vi "Clear-Receive.vi"(8 "错误输入":errorcluster caption="错误输入（无错误）", 10 "CANChannel":u32, 11 "DeviceType":T2=3 items=["PCI-CAN200"=7, "USB-CAN"=2, "USB-CAN200"=3]) -> (0 "错误输出":errorcluster, 1 "VCI_CAN_OBJ_R":T1={"ID"=96, 0, 0, 0, "TimeStamp"=0, "TimeFlag"=0, "SendType"=0, "RemoteFlag"=0, "ExternFlag"=0, "DataLen"=8, "Byte0"=0, "Byte1"=248, "Byte2"=17, "Byte3"=0, "Byte4"=0, "Byte5"=0, "Byte6"=0, "Byte7"=0, "Channel"=0, 77, 32} {"Byte7" format="%x"; "Byte6" format="%x"; "Byte5" format="%x"; "Byte4" format="%x"; "Byte3" format="%x"; "Byte2" format="%x"; "Byte1" format="%x"; "Byte0" format="%x"}, 2 "Result":bool=TRUE, 3 "DeviceTypeOut":u16(ring)=7 items=["PCI-CAN200"=7], 4 "帧数据":string, 5 "每次接收完时间":u32, 6 "data":string, 7 "ErrorSource":string)   [LabVIEW 2013]
uses:
  DevType.ctl
  VCI_CAN.dll
panel:
  out "VCI_CAN_OBJ_R 2":T1
  out "长度":string
  out "帧ID":string
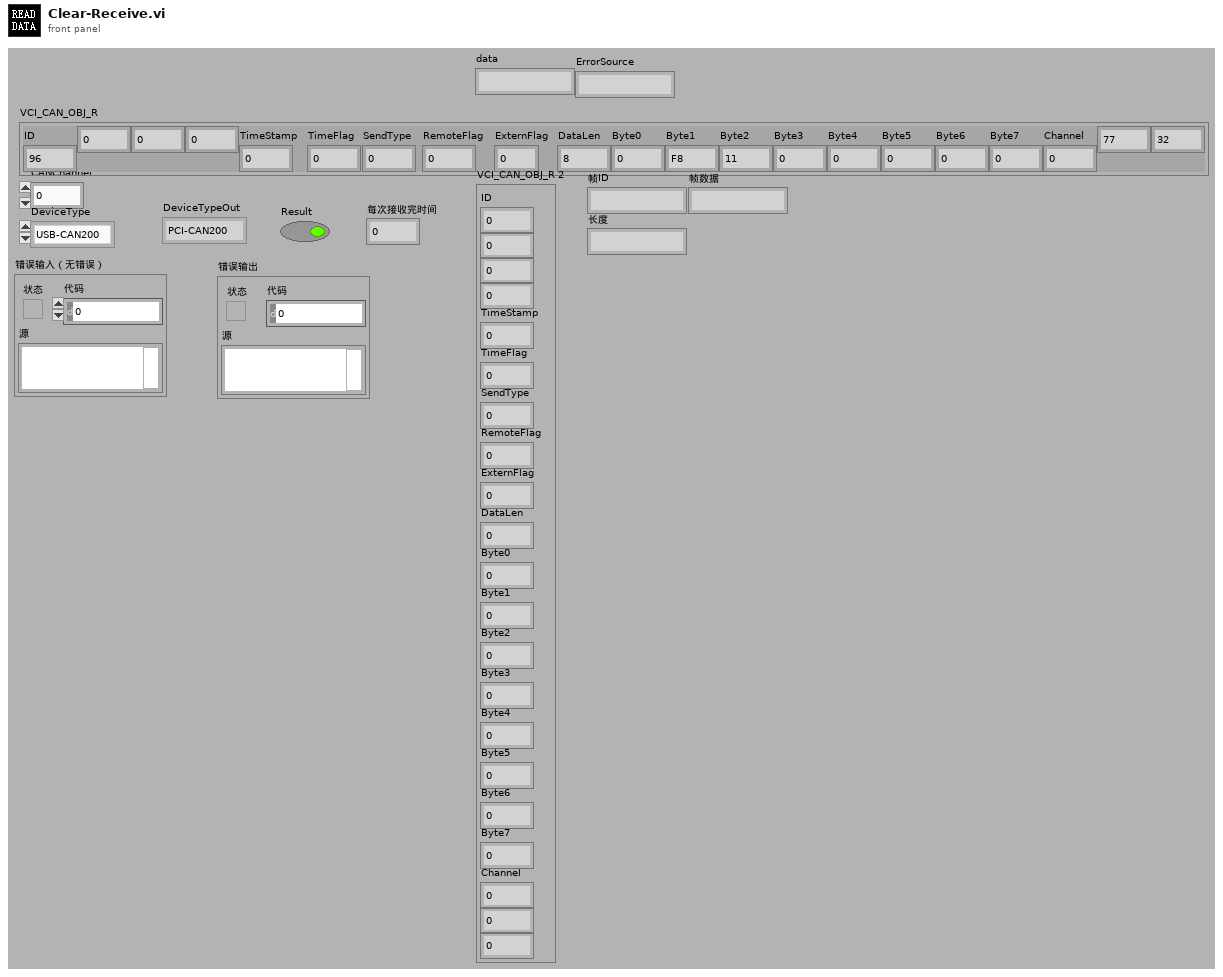
[diagram p1: front panel]
types:
  T1 = cluster{"ID":u8, u8, u8, u8, "TimeStamp":u32, "TimeFlag":u8, "SendType":u8, "RemoteFlag":u8, "ExternFlag":u8, "DataLen":u8, "Byte0":u8, "Byte1":u8, "Byte2":u8, "Byte3":u8, "Byte4":u8, "Byte5":u8, "Byte6":u8, "Byte7":u8, "Channel":u8, u8, u8}
  T2 = typedef "DevType.ctl" = u16
  T3 = cluster{"ID":u8, u8, u8, u8, "TimeStamp":u32, "TimeFlag":u8, "SendType":u8, "RemoteFlag":u8, "ExternFlag":u8, "DataLen":u8, u8, u8, u8, u8, u8, u8, u8, u8, u8, u8, u8}
  T4 = cluster{"ID":u8, u8, u8, u8, "TimeStamp":u32, "TimeFlag":u8, "SendType":u8, "RemoteFlag":u8, "ExternFlag":u8, "DataLen":u8, u8, u8, u8, u8, u8, u8, u8, u8, u8, u8, u8}[]
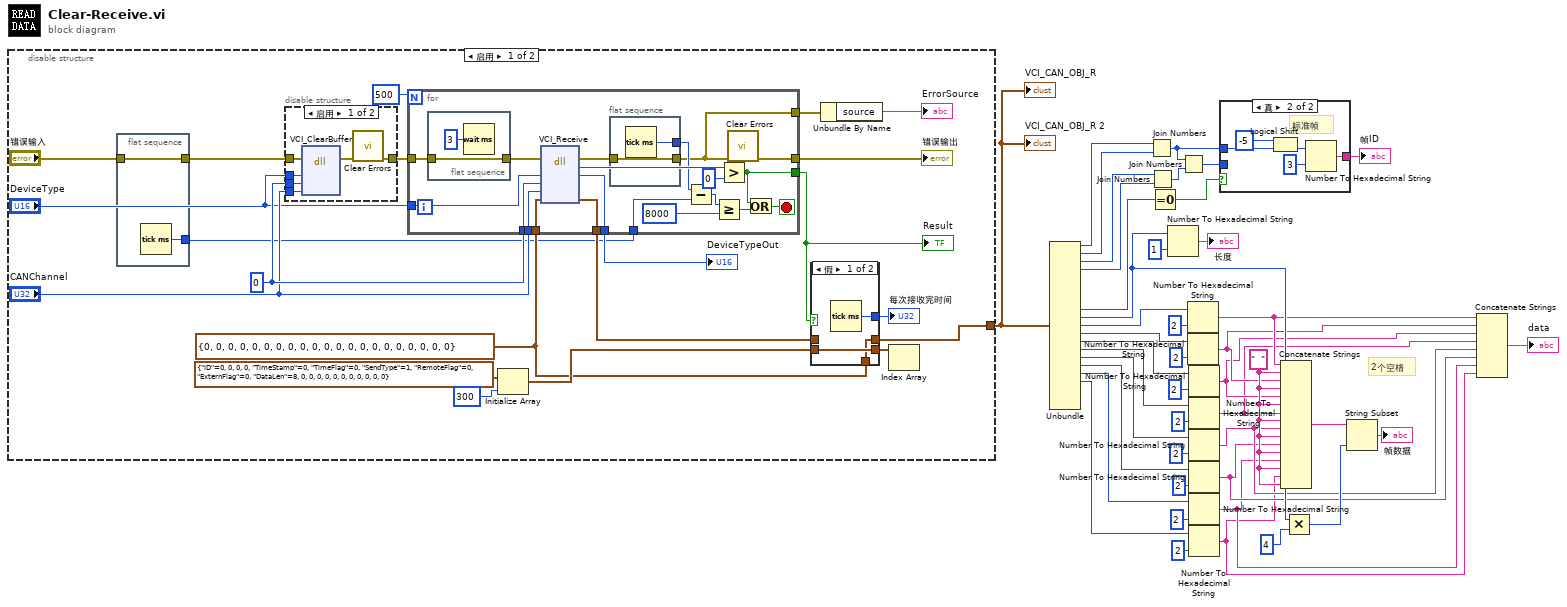
[diagram p0: block diagram]
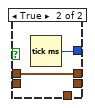
[diagram p3: hidden frame]
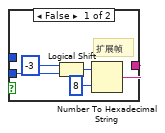
[diagram p5: hidden frame]
diagram:
  w23 = "  " ("字符串")
  # "2个空格"
  n1 = disable-structure shown="启用" {
    disable-tunnel: [w51 _] -> w10
    frame Enabled {
      w52 = T1 {"ID"=0, 0, 0, 0, "TimeStamp"=0, "TimeFlag"=0, "SendType"=0, "RemoteFlag"=0, "ExternFlag"=0, "DataLen"=0, "Byte0"=0, "Byte1"=0, "Byte2"=0, "Byte3"=0, "Byte4"=0, "Byte5"=0, "Byte6"=0, "Byte7"=0, "Channel"=0, 0, 0} ("VCI_CAN_OBJ_R 2")
      w64 = 0
      n2 = flat-sequence {
        tunnel: [w67] -> w50
        tunnel: "错误输入" -> [w67]
        tunnel: [w66] -> w47
        frame #0 {
          n3 = Tick Count (ms)() -> (millisecond timer value=w66:u32)
        }
      }
      n4 = disable-structure shown="启用" {
        disable-tunnel: w50 -> [w73 w74]
        disable-tunnel: w64 -> [w72 _]
        disable-tunnel: [w68 w74] -> w63
        disable-tunnel: "CANChannel" -> [w70 _]
        disable-tunnel: "DeviceType" -> [w69 _]
        frame Enabled {
          n5 = dll-call lib="PTH1rabs E桌面江淮测试*海马五菱长丰江淮长安TBOX20181103InstrumentDriversUSB-CANVCI_CAN.dll" fn="VCI_ClearBuffer"(error in=w73, "DeviceType"=w69, "DeviceInd"=w72, "CANInd"=w70) -> (error out=w71:errorcluster)  [unwired: 6 in, 1 out]
          n6 = call <vilib>:"Clear Errors.vi"("error in (no error)"=w71) -> ("error out"=w68:errorcluster)  [unwired: 6 in]
        }
        frame Disabled {
        }
      }
      n7 = for {
        N: 500 -> [_]
        tunnel: [w93] -> w65
        tunnel: "DeviceType" -> [w92]
        tunnel: w64 -> [w91]
        tunnel: "CANChannel" -> [w88]
        tunnel: [w78] -> w61
        tunnel: [w87] -> w60
        tunnel: w52 -> [w86]
        tunnel: w47 -> [w82]
        tunnel: [w75] -> w46
        tunnel: w63 -> [w90]
        tunnel: [w76] -> w48
        stop <- w77 stop-if-true
        n8 = flat-sequence {
          tunnel: w90 -> [w97]
          tunnel: [w97] -> w89
          frame #0 {
            n9 = Wait (ms)(milliseconds to wait=u32 3 ("等待时间（毫秒）")) -> ()  [unwired: 1 out]
          }
        }
        n10 = dll-call lib="PTH1rabs E桌面江淮测试*海马五菱长丰江淮长安TBOX20181103InstrumentDriversUSB-CANVCI_CAN.dll" fn="VCI_Receive"(error in=w89, "DeviceType"=w92, "DeviceInd"=w91, "CANInd"=w88, "VCI_CAN_OBJ_R"=w86) -> (error out=w85:errorcluster, "返回类型"=w94:u32, "DeviceType"=w93:u32, "VCI_CAN_OBJ_R"=w87:T1)  [unwired: 4 in, 1 out]
        n11 = flat-sequence {
          tunnel: w85 -> [w96]
          tunnel: [w96] -> w75
          tunnel: [w95] -> w83
          frame #0 {
            n12 = Tick Count (ms)() -> (millisecond timer value=w95:u32)
          }
        }
        n13 = Subtract(x=w83, y=w82) -> (x-y=w81:u32)
        n14 = Greater Or Equal?(x=w81, y=8000) -> (x >= y?=w79:bool)
        n15 = Greater?(x=w94, y=u32 0) -> (0:w78:bool)
        n16 = call <vilib>:"Clear Errors.vi"("error in (no error)"=w75) -> ("error out"=w76:errorcluster)  [unwired: 6 in]
        n17 = Or(x=w78, y=w79) -> (x .or. y?=w77:bool)
      }
      "错误输出" <- w48
      "Result" <- w61
      "DeviceTypeOut" <- w65
      n18 = Initialize Array(T3 {"ID"=0, 0, 0, 0, "TimeStamp"=0, "TimeFlag"=0, "SendType"=1, "RemoteFlag"=0, "ExternFlag"=0, "DataLen"=8, 0, 0, 0, 0, 0, 0, 0, 0, 0, 0, 0} ("VCI_CAN_OBJ_R 2"), 300 ("维数大小")) -> (w53:T4)
      n19 = case shown="假" w61 {
        tunnel: w60 -> [_ w102]
        tunnel: [w101 _] -> w54
        tunnel: w53 -> [w101 _]
        tunnel: [w100 w103] -> w59
        tunnel: [w99 w102] -> w51
        tunnel: w52 -> [w99 _]
        frame False {
          n20 = Tick Count (ms)() -> (millisecond timer value=w100:u32)
        }
        frame True {
          n21 = Tick Count (ms)() -> (millisecond timer value=w103:u32)
        }
      }
      "每次接收完时间" <- w59
      n22 = Unbundle By Name(w46) -> ("source"=→"ErrorSource":string)
      n23 = Index Array(array=w54) -> ()  [unwired: 1 in, 1 out]
    }
    frame Disabled {
    }
  }
  "VCI_CAN_OBJ_R" <- w10
  "VCI_CAN_OBJ_R 2" <- w10
  n24 = Unbundle(w10) -> ("ID"=w43:u8, w44:u8, w42:u8, w41:u8, "ExternFlag"=w18:u8, "DataLen"=w22:u8, "Byte0"=w40:u8, "Byte1"=w39:u8, "Byte2"=w37:u8, "Byte3"=w36:u8, "Byte4"=w35:u8, "Byte5"=w34:u8, "Byte6"=w33:u8, "Byte7"=w32:u8)  [unwired: 7 out]
  n25 = Join Numbers(hi=w43, lo=w44) -> ((hi.lo)=w14:u16)
  n26 = Join Numbers(hi=w42, lo=w41) -> ((hi.lo)=w15:u16)
  n27 = Equal To 0?(x=w18) -> (x = 0?=w17:bool)
  n28 = Number To Hexadecimal String(1:i16 1 ("宽度(-)"), 2:w22) -> (0:→"长度":string)
  n29 = Join Numbers(hi=w14, lo=w15) -> ((hi.lo)=w16:u32)
  n30 = Number To Hexadecimal String(1:i16 2 ("宽度(-)"), 2:w40) -> (0:w9:string)
  n31 = Number To Hexadecimal String(1:i16 2 ("宽度(-)"), 2:w39) -> (0:w8:string)
  n32 = Number To Hexadecimal String(1:i16 2 ("宽度(-)"), 2:w37) -> (0:w7:string)
  n33 = Number To Hexadecimal String(1:i16 2 ("宽度(-)"), 2:w36) -> (0:w6:string)
  n34 = Number To Hexadecimal String(1:i16 2 ("宽度(-)"), 2:w35) -> (0:w5:string)
  n35 = Number To Hexadecimal String(1:i16 2 ("宽度(-)"), 2:w34) -> (0:w4:string)
  n36 = Number To Hexadecimal String(1:i16 2 ("宽度(-)"), 2:w33) -> (0:w3:string)
  n37 = Number To Hexadecimal String(1:i16 2 ("宽度(-)"), 2:w32) -> (0:w2:string)
  n38 = case shown="真" w17 {
    tunnel: [w107 w110] -> w13
    tunnel: w16 -> [w105 _]
    tunnel: w14 -> [_ w109]
    frame False {
      # "扩展帧"
      n39 = Logical Shift(y=i8 -3, x=w105) -> (x << y=w106:u32)
      n40 = Number To Hexadecimal String(1:i16 8 ("宽度(-)"), 2:w106) -> (0:w107:string)
    }
    frame True {
      # "标准帧"
      n41 = Logical Shift(y=i8 -5, x=w109) -> (x << y=w112:u16)
      n42 = Number To Hexadecimal String(1:i16 3 ("宽度(-)"), 2:w112) -> (0:w110:string)
    }
  }
  "帧ID" <- w13
  n43 = Concatenate Strings(w9, w23, w8, w23, w7, w23, w6, w23, w5, w23, w4, w23, w3, w23, w2, w23) -> (w19:string)
  n44 = Multiply(x=w22, y=u8 4) -> (x*y=w20:u8)
  n45 = String Subset(string=w19, length (rest)=w20) -> (substring=→"帧数据":string)  [unwired: 1 in]
  n46 = Concatenate Strings(w9, w8, w7, w6, w5, w4, w3, w2) -> (→"data":string)
